vi "Remove Emptys From String Array.vi"(11 "Array in":string[](array[string])) -> (3 "Array out":string[](array[string]))   [LabVIEW 2017, in "CSM Shared.lvlib"]
uses:
  CSM Shared.lvlib
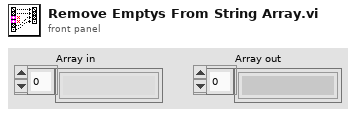
[diagram p1: front panel]
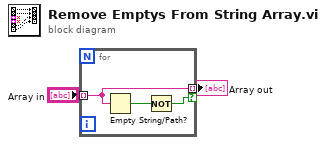
[diagram p0: block diagram]
diagram:
  n1 = for {
    tunnel: [w5] -> w1 mode=indexing if=w3
    tunnel: "Array in" -> [w5] mode=indexing
    n2 = Empty String/Path?(string/path=w5) -> (empty?=w4:bool)
    n3 = Not(x=w4) -> (.not. x?=w3:bool)
  }
  "Array out" <- w1
